vi "Fetch (Measurements).vi"(0 "VISA resource name":refnum<visa-resource-name>, 5 "Timeout (10000 ms)":i32=10000 format="%#.6g", 11 "error in (no error)":errorcluster) -> (3 "Voltage":sgl[](array[numeric]), 4 "VISA resource name out":refnum<visa-resource-name>, 6 "Current":sgl[](array[numeric]), 8 "Resistance":sgl[](array[numeric]), 10 "Timestamp":sgl[](array[numeric]), 14 "Status":sgl[](array[numeric]), 15 "error out":errorcluster)   [LabVIEW 2009, in "Keithley 24XX.lvlib"]
doc: "Fetches data for voltage, current, resistance, timestamp, and status. These readings are then provided in separate arrays for each type of reading.\n\n<B>Note</B> Use this VI only with other low-level VIs. The high-level VIs automatically incorporate this functionality. This VI does not check the instrument status. If you want to check the instrument status, call the Error Query VI at the conclusion of the sequence."
uses:
  <instrlib>/Keithley 24XX/Keithley 24XX.lvlib
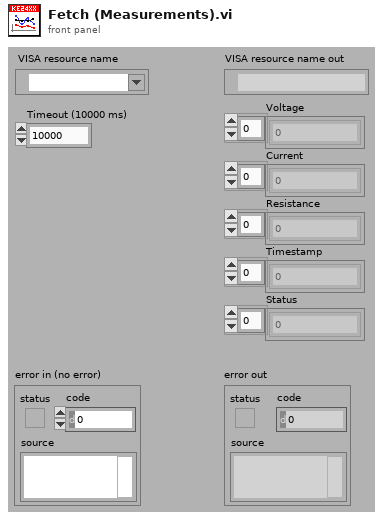
[diagram p1: front panel]
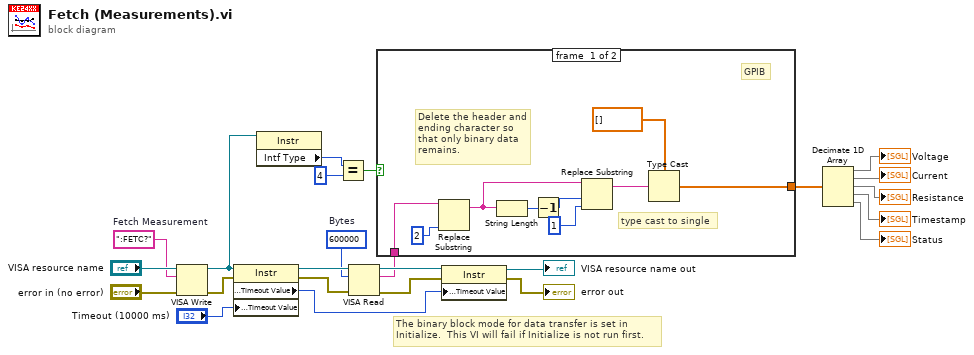
[diagram p0: block diagram]
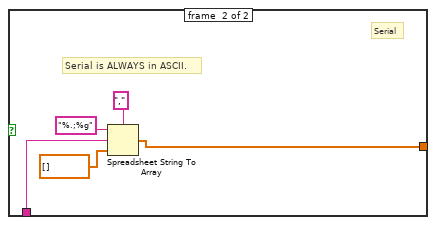
[diagram p2: hidden frame]
diagram:
  w22 = ":FETC?"  # Fetch Measurement
  w12 = u32 600000  # Bytes
  # "The binary block mode for data transfer is set in Initialize.  This VI will fail if Initialize is not run first."
  n1 = VISA Write(VISA resource name="VISA resource name", write buffer=w22, error in (no error)="error in (no error)") -> (VISA resource name out=w4:refnum<visa-resource-name>, error out=w21:errorcluster)  [unwired: 1 out]
  n2 = property class="Instr"(reference=w4, error in=w21, "General Settings:Timeout Value"="Timeout (10000 ms)") -> (reference out=w20:refnum<visa-resource-name>, error out=w19:errorcluster, "General Settings:Timeout Value"=w15:u32)
  n3 = property class="Instr"(reference=w4) -> ("Intf Type"=w3:u16)  [unwired: 1 in, 2 out]
  n4 = Equal?(x=w3, y=u16 4) -> (x = y?=w1:bool)
  n5 = VISA Read(VISA resource name=w20, byte count=w12, error in (no error)=w19) -> (VISA resource name out=w17:refnum<visa-resource-name>, read buffer=w11:string, error out=w16:errorcluster)  [unwired: 1 out]
  n6 = case shown="False" w1 {
    tunnel: w11 -> [w33 w38]
    tunnel: [w25 w34] -> w10
    frame #0 {
      # "Delete the header and ending character so that only binary data remains."
      # "GPIB"
      # "type cast to single"
      n7 = Replace Substring(2:2 ("length (len. of substring)"), 5:w33) -> (1:w31:string)  [unwired: 2 in, 1 out]
      n8 = String Length(string=w31) -> (length=w30:i32)
      n9 = Decrement(x=w30) -> (x-1=w29:i32)
      n10 = Replace Substring(2:1 ("length (len. of substring)"), 3:w29, 5:w31) -> (1:w27:string)  [unwired: 1 in, 1 out]
      n11 = Type Cast(type=sgl[] [], x=w27) -> (*(type *) &x=w25:sgl[])
    }
    frame #1 {
      # "Serial is ALWAYS in ASCII."
      # "Serial"
      n12 = Spreadsheet String To Array(delimiter (Tab)=",", format string="%.;%g", spreadsheet string=w38, array type (2D Dbl)=sgl[] []) -> (array=w34:sgl[])
    }
  }
  n13 = property class="Instr"(reference=w17, error in=w16, "General Settings:Timeout Value"=w15) -> (reference out=→"VISA resource name out":refnum<visa-resource-name>, error out=→"error out":errorcluster)
  n14 = Decimate 1D Array(w10) -> (→"Voltage":sgl[], →"Current":sgl[], →"Resistance":sgl[], →"Timestamp":sgl[], →"Status":sgl[])
